vi "IPVoice.FrameReader.vi"(7 "timeout (10sec)":u32=2000 caption="超时（10秒）", 8 "error in (no error)":errorcluster caption="错误输入（无错误）", 10 "Frame CMD":T1(ring), 11 "FrameReader Port":refnum<visa-resource-name> caption="VISA资源名称") -> (0 "错误输出":errorcluster, 1 "写入命令":u8[](array[numeric]) format="%02x", 2 "读取缓冲区":string, 3 "OK?":bool)   [LabVIEW 2012, in "Lib_UEL.ATE.lvlib" / "Lib_IPVoice.lvlib"]
uses:
  Lib_IPVoice.lvlib
  <vilib>/Instr/_visa.llb/VISA Configure Serial Port (Instr).vi
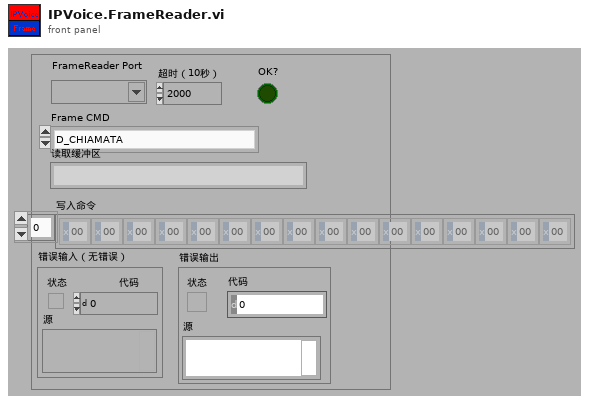
[diagram p1: front panel]
types:
  T1 = enum16{"D_CHIAMATA", "TEST_FRAME", "D_INGRESSO_IN_TEST", "D_FONIA", "C_CHIAMATA"}
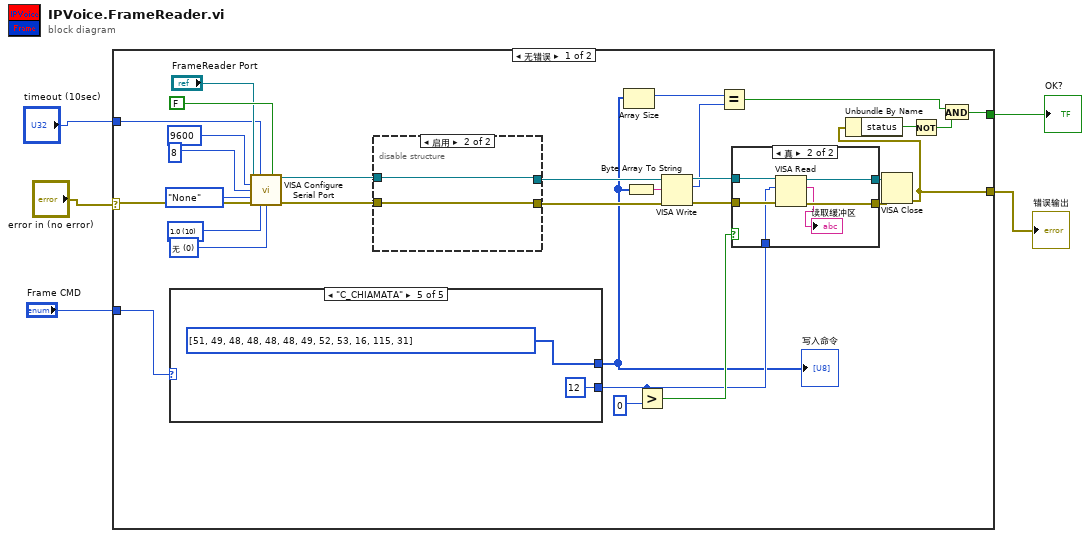
[diagram p0: block diagram]
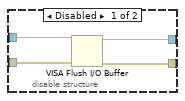
[diagram p2: hidden frame]
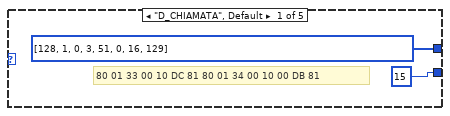
[diagram p4: hidden frame]
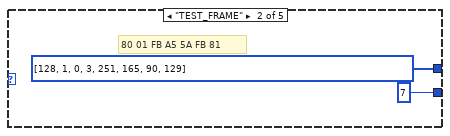
[diagram p5: hidden frame]
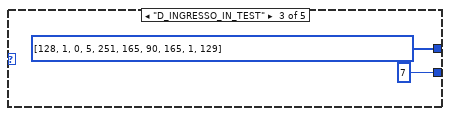
[diagram p6: hidden frame]
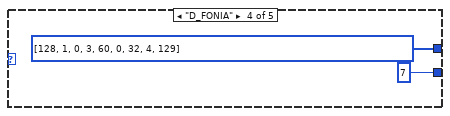
[diagram p7: hidden frame]
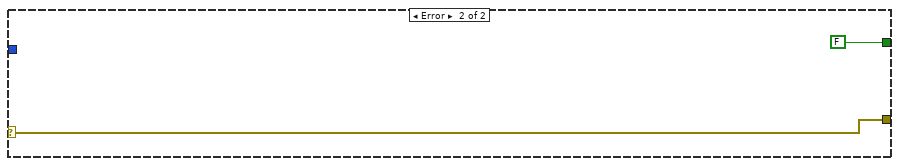
[diagram p8: hidden frame]
diagram:
  n1 = case shown="无错误" "error in (no error)" {
    selector: "error in (no error)" -> [w27 w61]
    tunnel: "Frame CMD" -> [w28 _]
    tunnel: [w10 w61] -> w3
    tunnel: "timeout (10sec)" -> [w18 _]
    tunnel: [w8 FALSE] -> w1
    frame No Error {
      w35 = u16 0 items=["无", "XON/XOFF", "RTS/CTS", "XON/XOFF & RTS/CTS", "DTR/DSR", "XON/XOFF & DTR/DSR"] ("flow control (0:none)")
      w34 = u16 10 items=["1.0"=10, "1.5"=15, "2.0"=20] ("stop bits (10: 1 bit)")
      n2 = case shown="\"C_CHIAMATA\"" w28 {
        tunnel: [u8[] [128, 1, 0, 3, 51, 0, 16, 129] ("无符号字节数组") u8[] [128, 1, 0, 3, 251, 165, 90, 129] ("无符号字节数组") u8[] [128, 1, 0, 5, 251, 165, 90, 165, 1, 129] ("无符号字节数组") u8[] [128, 1, 0, 3, 60, 0, 32, 4, 129] ("无符号字节数组") u8[] [51, 49, 48, 48, 48, 48, 49, 52, 53, 16, 115, 31] ("无符号字节数组")] -> w11
        tunnel: [15 ("y") 7 7 7 12 ("y")] -> w22
        frame "D_CHIAMATA", Default {
          # "80 01 33 00 10 DC 81 80 01 34 00 10 00 DB 81"
        }
        frame "TEST_FRAME" {
          # "80 01 FB A5 5A FB 81"
        }
        frame "D_INGRESSO_IN_TEST" {
        }
        frame "D_FONIA" {
        }
        frame "C_CHIAMATA" {
        }
      }
      "写入命令" <- w11
      n3 = call-poly "VISA Configure Serial Port"("VISA resource name"="FrameReader Port", "timeout (10sec)"=w18, "Enable Termination\nChar (T)"=FALSE ("Disable Termination\nChar (T)"), "baud rate (9600)"=u32 9600, "data bits (8)"=u16 8, "parity (0:none)"=enum16{"None", "Odd", "Even", "Mark", "Space"}."None", "error in (no error)"=w27, "stop bits (10: 1 bit)"=w34, "flow control (0:none)"=w35) -> ("VISA resource name out"=w17:refnum<visa-resource-name>, "error out"=w16:errorcluster)  [unwired: 5 in]
      n4 = disable-structure shown="启用" {
        disable-tunnel: w17 -> [w39 w41]
        disable-tunnel: w16 -> [w38 w40]
        disable-tunnel: [w37 w41] -> w15
        disable-tunnel: [w36 w40] -> w14
        frame Disabled {
          n5 = VISA Flush I/O Buffer(VISA resource name=w39, error in (no error)=w38) -> (VISA resource name out=w37:refnum<visa-resource-name>, error out=w36:errorcluster)  [unwired: 1 in]
        }
        frame Enabled {
        }
      }
      n6 = Array Size(array=w11) -> (size(s)=w13:i32)
      n7 = Byte Array To String(unsigned byte array=w11) -> (string=w26:string)
      n8 = Greater?(x=w22, y=0) -> (0:w23:bool)
      n9 = VISA Write(VISA resource name=w15, write buffer=w26, error in (no error)=w14) -> (VISA resource name out=w24:refnum<visa-resource-name>, return count=w12:u32, error out=w25:errorcluster)
      n10 = Equal?(x=w13, y=w12) -> (x = y?=w6:bool)
      n11 = case shown="真" w23 {
        tunnel: w25 -> [w42 w49]
        tunnel: w24 -> [w43 w48]
        tunnel: w22 -> [_ w47]
        tunnel: [w43 w46] -> w21
        tunnel: [w42 w45] -> w20
        frame False {
        }
        frame True {
          n12 = VISA Read(VISA resource name=w48, byte count=w47, error in (no error)=w49) -> (VISA resource name out=w46:refnum<visa-resource-name>, read buffer=→"读取缓冲区":string, error out=w45:errorcluster)  [unwired: 1 out]
        }
      }
      n13 = VISA Close(VISA resource name=w21, error in (no error)=w20) -> (error out=w10:errorcluster)
      n14 = Unbundle By Name(w10) -> ("status"=w9:bool)
      n15 = Not(x=w9) -> (.not. x?=w7:bool)
      n16 = And(x=w6, y=w7) -> (x .and. y?=w8:bool)
    }
    frame Error {
    }
  }
  "错误输出" <- w3
  "OK?" <- w1
